vi "Write Data.vi"(8 "error in (no error)":errorcluster, 9 "Publication Time":timestamp, 10 "Value":variant, 11 "MCListboxItemNamesBinding In":refnum<class "MCListboxItemNamesBinding.lvclass">) -> (0 "error out":errorcluster, 3 "MCListboxItemNamesBinding Out":refnum<class "MCListboxItemNamesBinding.lvclass">)   [LabVIEW 2015, in "Transport.lvlib" / "MCListboxItemNamesBinding.lvclass"]
doc: "<License>\nCopyright © 2017 Composed Systems, LLC | All rights reserved\nwww.composed.io\n\nAuthor: Ethan Stern <ethan.stern@composed.io>\n\nThis software is provided \"AS IS\" WITHOUT WARRANTIES, either express or implied, AND IS FOR EDUCATIONAL PURPOSES ONLY.\n</License>"
uses:
  MCListboxItemNamesBinding.lvclass
  MCListboxItemNamesBinding.lvclass/MCListboxItemNamesBinding.ctl
  <vilib>/Utility/miscctls.llb/LVRowAndColumnUnsignedTypeDef.ctl
  <vilib>/Utility/error.llb/Error Cluster From Error Code.vi
  <vilib>/ErrorRing/Error Ring.xnode
  <vilib>/Utility/Data Type/NI_Data Type.lvlib
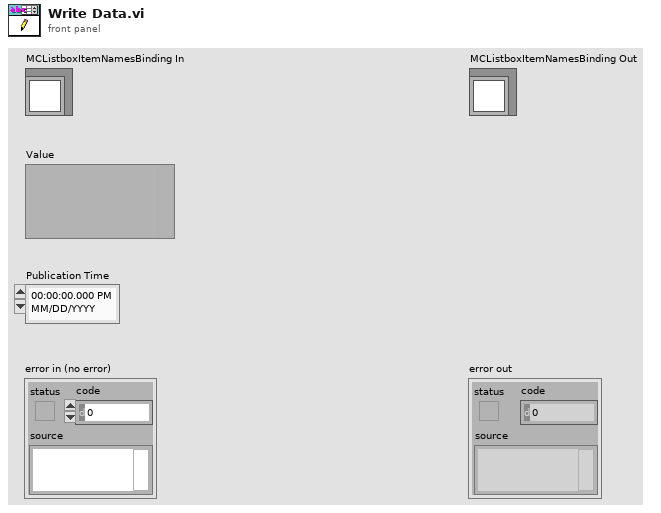
[diagram p1: front panel]
types:
  T1 = typedef "Transport.lvlib/MCListboxItemNamesBinding.lvclass/MCListbox Binding Options.ctl" = bool
  T2 = typedef "LVRowAndColumnUnsignedTypeDef.ctl" = cluster{"Row":u32, "Column":u32}
  T3 = typedef "NI_Data Type.lvlib/Data Type.ctl" = enum8{"Invalid Type", "Void", "I8", "I16", "I32", "I64", "U8", "U16", "U32", "U64", "Single Float", "Double Float", "Extended Float", "Single Complex", "Double Complex", "Extended Complex", "Enum U8", "Enum U16", "Enum U32", "Enum U64", "Single Float With Unit", "Double Float With Unit", "Extended Float With Unit", "Single Complex with Unit", "Double Complex with Unit", "Extended Complex with Unit", "Boolean", "String", "Path", "Picture", "Tag", "Array", "Cluster", "Variant", "LV Variant", "Waveform", "Timestamp", "Digital Waveform", "Digital Data", "ExpressData", "Refnum", "External Data", "VI", "Poly VI", "LabVIEW Class Instance", "Fixed Point"}
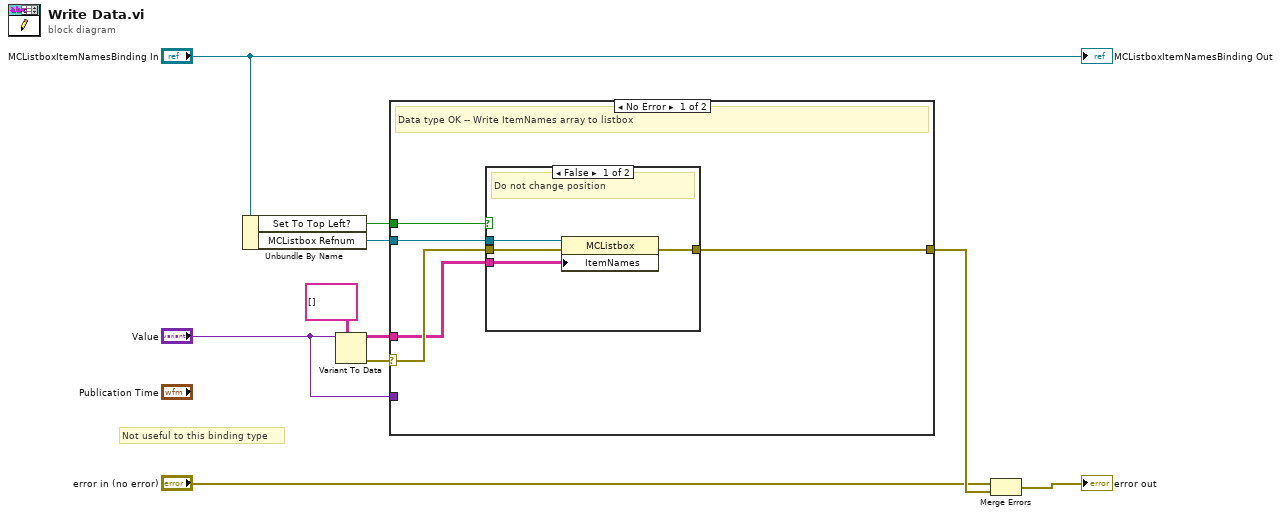
[diagram p0: block diagram]
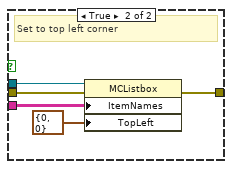
[diagram p2: hidden frame]
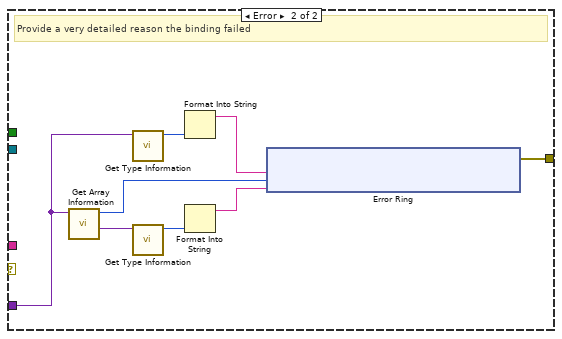
[diagram p3: hidden frame]
diagram:
  # "Not useful to this binding type"
  n1 = Unbundle By Name("MCListboxItemNamesBinding In") -> ("Set To Top Left?"=w3:T1, "MCListbox Refnum"=w4:refnum<vi>)
  n2 = Variant To Data(type=string[][] [], Variant="Value") -> (data=w5:string[][], error out=w6:errorcluster)  [unwired: 1 in]
  n3 = case shown="No Error" w6 {
    selector: w6 -> [w14 _]
    tunnel: w5 -> [w13 _]
    tunnel: w4 -> [w15 _]
    tunnel: "Value" -> [_ w29]
    tunnel: w3 -> [w11 _]
    tunnel: [w12 w32] -> w10
    frame No Error {
      # "Data type OK -- Write ItemNames array to listbox"
      n4 = case shown="False" w11 {
        tunnel: w15 -> [w19 w24]
        tunnel: w14 -> [w18 w23]
        tunnel: w13 -> [w16 w22]
        tunnel: [w17 w21] -> w12
        frame False {
          # "Do not change position"
          n5 = property class="MCListbox"(reference=w19, error in=w18, "ItemNames"=w16) -> (error out=w17:errorcluster)  [unwired: 1 out]
        }
        frame True {
          # "Set to top left corner"
          n6 = property class="MCListbox"(reference=w24, error in=w23, "ItemNames"=w22, "TopLeft"=T2 {"Row"=0, "Column"=0} ("Top Left Visible Cell")) -> (error out=w21:errorcluster)  [unwired: 1 out]
        }
      }
    }
    frame Error {
      # "Provide a very detailed reason the binding failed"
      n7 = call <vilib>:"Get Array Information.vi"("Variant"=w29) -> ("Array Element Data Type"=w31:variant, "Number of Dimensions"=w26:i32)  [unwired: 7 in, 2 out]
      n8 = call <vilib>:"Get Type Information.vi"("Variant"=w29) -> ("Type"=w28:T3)  [unwired: 6 in, 4 out]
      n9 = call <vilib>:"Get Type Information.vi"("Variant"=w31) -> ("Type"=w30:T3)  [unwired: 6 in, 4 out]
      n10 = Format Into String(w28) -> (resulting string=w27:string)  [unwired: 3 in, 1 out]
      n11 = Format Into String(w30) -> (resulting string=w25:string)  [unwired: 3 in, 1 out]
      n12 = xnode "Error Ring"("parameter 0"=w27, "parameter 1"=w26, "parameter 2"=w25) -> ("error out"=w32:errorcluster)
    }
  }
  n13 = Merge Errors("error in (no error)", w10) -> (→"error out":errorcluster)
  "MCListboxItemNamesBinding Out" <- "MCListboxItemNamesBinding In"
